vi "Login_Main P3.vi"() -> (3 "Login pass":bool)   [LabVIEW 2022 SP3]
uses:
  <vilib>/Utility/error.llb/Trim Whitespace One-Sided.vi
  Globals/Phase III Globals.vi
  <vilib>/Utility/file.llb/Read Delimited Spreadsheet (string).vi
  <vilib>/Utility/file.llb/Write Delimited Spreadsheet (string).vi
panel:
  in  "Enter":bool
  in  "Stop Button":bool
  out "Pass = True":bool
  in  "Change Password":bool
  in  "Show Password":bool
  in  "Password":string
  in  "Select User":u16(ring) items=["Vigneshwaran", "Kannan"]
  # "Agnikul Cosmos"
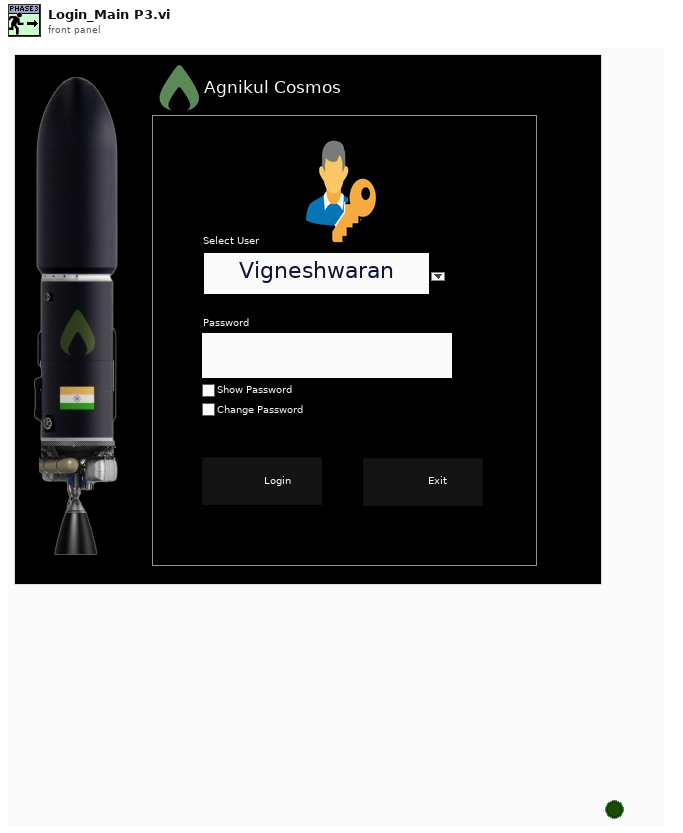
[diagram p1: front panel]
types:
  T1 = typedef "file folder ctl.ctl" = cluster{"Datalog path":path, "Configuration path":path, "Signal list path":path, "Sub vi's":path, "Authentication":path}
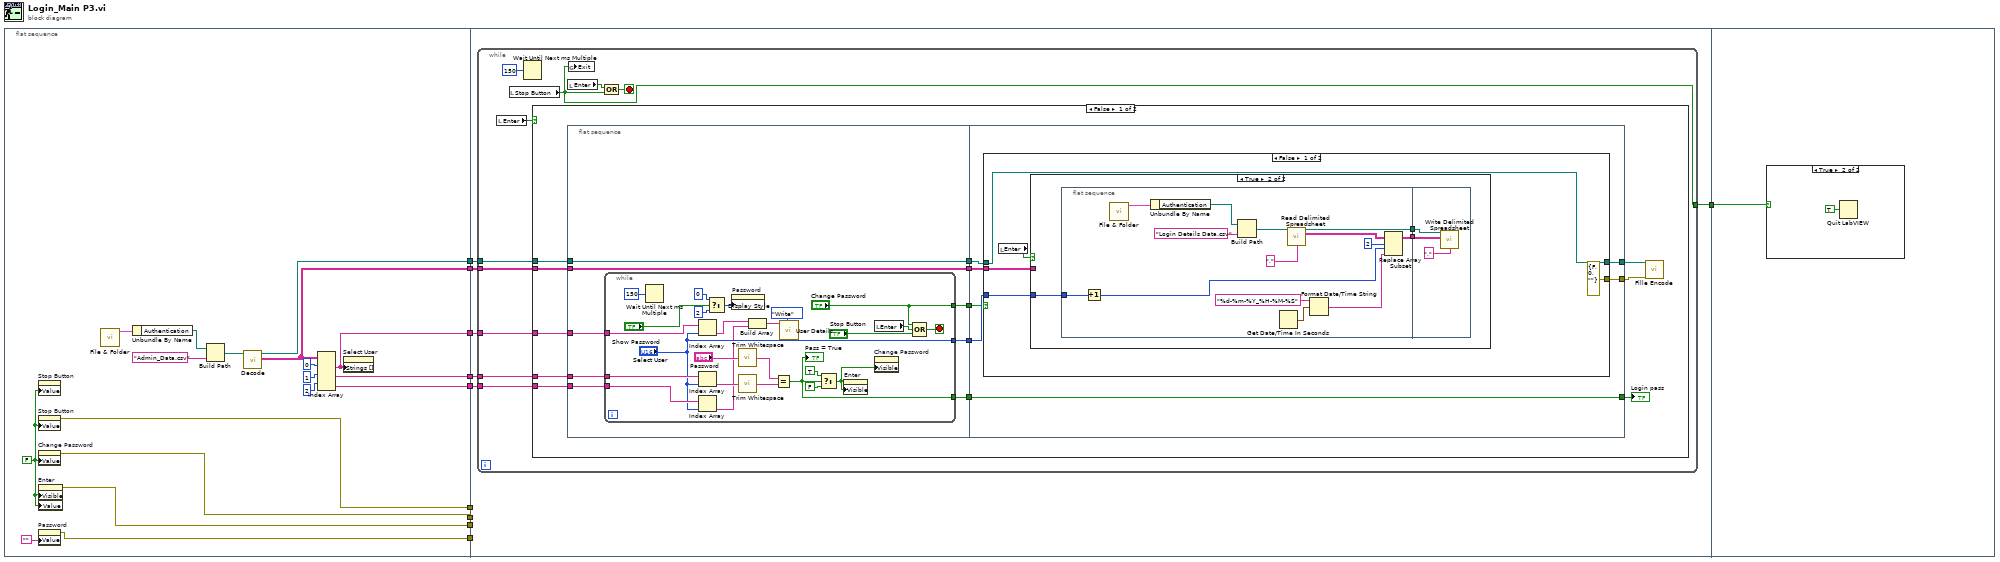
[diagram p0: block diagram]
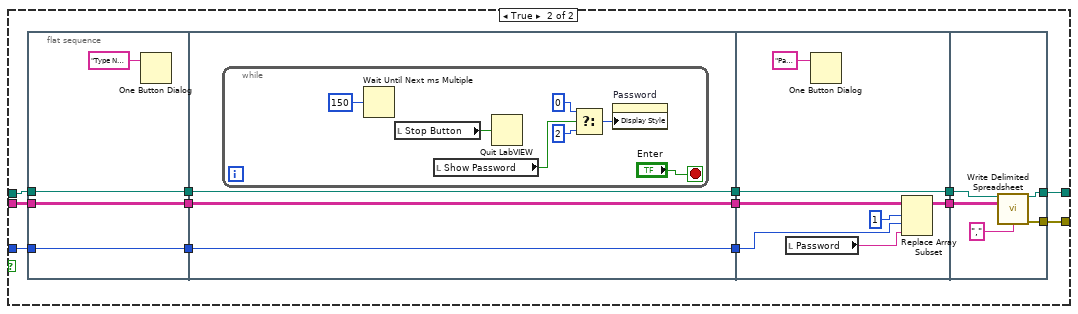
[diagram p3: hidden frame]
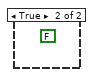
[diagram p4: hidden frame]
diagram:
  n1 = flat-sequence {
    tunnel: [w26] -> w10
    tunnel: [w11] -> w9
    tunnel: [w20] -> w8
    tunnel: [w25] -> w7
    tunnel: [w12] -> w6
    tunnel: [w22] -> w5
    tunnel: [w21] -> w4
    tunnel: [w19] -> w3
    tunnel: [w15] -> w2
    tunnel: w4 -> [_]
    tunnel: w5 -> [_]
    tunnel: w6 -> [w32]
    tunnel: w7 -> [_]
    tunnel: w8 -> [_]
    tunnel: w9 -> [w33]
    tunnel: w10 -> [w34]
    tunnel: w3 -> [w31]
    tunnel: w2 -> [w30]
    tunnel: [w29] -> w1
    tunnel: w1 -> [w162]
    frame #0 {
      w14 = FALSE ("Change Password")
      n2 = property on="Stop Button" class="Bool (strict)"("Value"=w14) -> ()  [unwired: 2 in, 2 out]
      n3 = property on="Stop Button" class="Bool (strict)"("Value"=w14) -> (error out=w21:errorcluster)  [unwired: 2 in, 1 out]
      n4 = property on="Change Password" class="Bool (strict)"("Value"=w14) -> (error out=w25:errorcluster)  [unwired: 2 in, 1 out]
      n5 = property on="Enter" class="Bool (strict)"("Visible"=w14, "Value"=w14) -> (error out=w20:errorcluster)  [unwired: 2 in, 1 out]
      n6 = property on="Password" class="Str"("Value"="") -> (error out=w22:errorcluster)  [unwired: 2 in, 1 out]
      n7 = call "File & Folder.vi"() -> ("File Output"=w18:T1)  [unwired: 10 in, 1 out]
      n8 = Unbundle By Name(w18) -> ("Authentication"=w17:path)
      n9 = Build Path(base path=w17, name or relative path="Admin_Data.csv" ("name")) -> (appended path=w13:path)
      n10 = call "Decode.vi"("Encoded  File"=w13) -> ("array"=w11:string[][], "Decoded File"=w12:path)  [unwired: 9 in]
      n11 = Index Array(array=w11, index (row) #1=0 ("index (row)"), index (row) #2=1 ("index (row)"), index (row) #3=2 ("disabled index (col)")) -> (element #1=w19:string[], element #2=w26:string[], element #3=w15:string[])  [unwired: 3 in]
      n12 = property on="Select User" class="Ring (strict)"("Strings []"=w19) -> ()  [unwired: 2 in, 2 out]
    }
    frame #1 {
      n13 = while {
        tunnel: w34 -> [w43]
        tunnel: w33 -> [w42]
        tunnel: w32 -> [w41]
        tunnel: w31 -> [w39]
        tunnel: w30 -> [w38]
        tunnel: [w35] -> w29
        stop <- w37 stop-if-true
        n14 = local read "Enter"() -> (w40:bool)
        n15 = local read "Stop Button"() -> (w35:bool)
        n16 = Wait Until Next ms Multiple(millisecond multiple=u32 150) -> ()  [unwired: 1 out]
        n17 = case shown="False" w40 {
          tunnel: w43 -> [w55 _]
          tunnel: w42 -> [w54 _]
          tunnel: w41 -> [w51 _]
          tunnel: w39 -> [w50 _]
          tunnel: w38 -> [w49 _]
          frame False {
            n18 = flat-sequence {
              tunnel: [w65] -> w57
              tunnel: [w64] -> w56
              tunnel: w54 -> [w65]
              tunnel: w55 -> [w63]
              tunnel: [w62] -> w53
              tunnel: [w61] -> w52
              tunnel: w51 -> [w61]
              tunnel: w50 -> [w60]
              tunnel: w49 -> [w59]
              tunnel: [w58] -> w48
              tunnel: w57 -> [w97]
              tunnel: w56 -> [w96]
              tunnel: w53 -> [w95]
              tunnel: w52 -> [w91]
              tunnel: w48 -> [w94]
              tunnel: [w94] -> w47
              tunnel: [w93] -> w46
              tunnel: [w92] -> w45
              frame #0 {
                n19 = while {
                  tunnel: ["Select User"] -> w64
                  tunnel: w63 -> [w90]
                  tunnel: ["Change Password"] -> w62
                  tunnel: w60 -> [w74]
                  tunnel: w59 -> [w73]
                  tunnel: [w70] -> w58
                  stop <- w79 stop-if-true
                  n20 = Wait Until Next ms Multiple(millisecond multiple=u32 150) -> ()  [unwired: 1 out]
                  n21 = Index Array(array=w74, index="Select User") -> (element=w68:string)
                  n22 = Index Array(array=w90, index="Select User") -> (element=w89:string)
                  n23 = Index Array(array=w73, index="Select User") -> (element=w67:string)
                  n24 = Select(t=u32 0 ("Display Style"), s="Show Password", f=u32 2 ("Display Style")) -> (s? t:f=w83:u32)
                  n25 = property on="Password" class="Str"("Display Style"=w83) -> ()  [unwired: 2 in, 2 out]
                  n26 = call <vilib>:"Trim Whitespace.vi"("string"="Password") -> ("trimmed string"=w85:string)  [unwired: 1 in]
                  n27 = call <vilib>:"Trim Whitespace.vi"("string"=w89) -> ("trimmed string"=w75:string)  [unwired: 1 in]
                  n28 = Build Array(w68, w67) -> (w66:string[])
                  n29 = Equal?(x=w85, y=w75) -> (x = y?=w70:bool)
                  "Pass = True" <- w70
                  n30 = call "User Details.vi"("Enum"=enum16{"Read", "Write"}."Write", "User details"=w66) -> ()  [unwired: 8 in, 2 out]
                  n31 = Select(t=TRUE, s=w70, f=FALSE ("Visible")) -> (s? t:f=w76:bool)
                  n32 = property on="Enter" class="Bool (strict)"("Visible"=w76) -> ()  [unwired: 2 in, 2 out]
                  n33 = local read "Enter"() -> (w77:bool)
                  n34 = property on="Change Password" class="Bool (strict)"("Visible"=w76) -> ()  [unwired: 2 in, 2 out]
                  n35 = Compound Arithmetic op=OR("Change Password", w77, "Stop Button") -> (w79:bool)
                }
              }
              frame #1 {
                n36 = case shown="False" w95 {
                  tunnel: w97 -> [w102 w133]
                  tunnel: w96 -> [w101 w130]
                  tunnel: w91 -> [w99 w125]
                  tunnel: [w99 w124] -> w93
                  tunnel: [errorcluster {"status"=FALSE, "code"=0, "source"=""} ("error out") w123] -> w92
                  frame False {
                    n37 = local read "Enter"() -> (w100:bool)
                    n38 = case shown="True" w100 {
                      tunnel: w102 -> [_ _]
                      tunnel: w101 -> [_ w105]
                      frame False {
                      }
                      frame True {
                        n39 = flat-sequence {
                          tunnel: w105 -> [w119]
                          tunnel: [w109] -> w104
                          tunnel: [w108] -> w103
                          tunnel: w104 -> [w121]
                          tunnel: w103 -> [w122]
                          frame #0 {
                            n40 = Increment(x=w119) -> (x+1=w112:u16)
                            n41 = call "File & Folder.vi"() -> ("File Output"=w115:T1)  [unwired: 10 in, 1 out]
                            n42 = Unbundle By Name(w115) -> ("Authentication"=w114:path)
                            n43 = Build Path(base path=w114, name or relative path="Login Details Data.csv" ("name")) -> (appended path=w111:path)
                            n44 = Get Date/Time In Seconds() -> (seconds since 1Jan1904=w106:timestamp)
                            n45 = call-poly <vilib>:"Read Delimited Spreadsheet.vi"("file path (dialog if empty)"=w111, "delimiter (\\t)"="," ("delimiter (\\t)")) -> ("new file path (Not A Path if cancelled)"=w108:path, "all rows"=w110:string[][])  [unwired: 8 in, 4 out]
                            n46 = Format Date/Time String(time format string (%c)="%d-%m-%Y_%H-%M-%S", seconds (now)=w106) -> (date/time string=w117:string)  [unwired: 1 in]
                            n47 = Replace Array Subset(array=w110, new element=w117, index (row)=2, index (col)=w112) -> (w109:string[][])
                          }
                          frame #1 {
                            n48 = call-poly <vilib>:"Write Delimited Spreadsheet.vi"("file path (dialog if empty)"=w122, "2D data"=w121, "delimiter (\\t)"="," ("delimiter (\\t)")) -> ()  [unwired: 11 in, 2 out]
                          }
                        }
                      }
                    }
                  }
                  frame True {
                    n49 = flat-sequence {
                      tunnel: [w139] -> w134
                      tunnel: w133 -> [w139]
                      tunnel: [w138] -> w131
                      tunnel: w130 -> [w138]
                      tunnel: [w137] -> w126
                      tunnel: w125 -> [w137]
                      tunnel: [w142] -> w135
                      tunnel: w134 -> [w142]
                      tunnel: [w141] -> w132
                      tunnel: w131 -> [w141]
                      tunnel: [w140] -> w127
                      tunnel: w126 -> [w140]
                      tunnel: w135 -> [w155]
                      tunnel: w132 -> [w153]
                      tunnel: [w151] -> w129
                      tunnel: [w150] -> w128
                      tunnel: w127 -> [w150]
                      tunnel: w129 -> [w161]
                      tunnel: w128 -> [w160]
                      tunnel: [w158] -> w124
                      tunnel: [w157] -> w123
                      frame #0 {
                        n50 = One Button Dialog(message="Type New Password and Press Enter button") -> ()  [unwired: 1 in, 1 out]
                      }
                      frame #1 {
                        n51 = while {
                          stop <- "Enter" stop-if-true
                          n52 = Wait Until Next ms Multiple(millisecond multiple=u32 150) -> ()  [unwired: 1 out]
                          n53 = local read "Stop Button"() -> (w148:bool)
                          n54 = local read "Show Password"() -> (w143:bool)
                          n55 = Quit LabVIEW(quit? (T)=w148) -> ()
                          n56 = Select(t=u32 0 ("Display Style"), s=w143, f=u32 2 ("Display Style")) -> (s? t:f=w144:u32)
                          n57 = property on="Password" class="Str"("Display Style"=w144) -> ()  [unwired: 2 in, 2 out]
                        }
                      }
                      frame #2 {
                        n58 = local read "Password"() -> (w152:string)
                        n59 = One Button Dialog(message="Password changed successfully, Please Login with new Password") -> ()  [unwired: 1 in, 1 out]
                        n60 = Replace Array Subset(array=w155, new element=w152, index (row)=1, index (col)=w153) -> (w151:string[][])
                      }
                      frame #3 {
                        n61 = call-poly <vilib>:"Write Delimited Spreadsheet.vi"("file path (dialog if empty)"=w160, "2D data"=w161, "delimiter (\\t)"="," ("delimiter (\\t)")) -> ("new file path (Not A Path if cancelled)"=w158:path, "error out"=w157:errorcluster)  [unwired: 11 in]
                      }
                    }
                  }
                }
              }
            }
            n62 = call "Fille Encode.vi"("error in"=w45, "Original File"=w46) -> ()  [unwired: 8 in, 2 out]
            "Login pass" <- w47
          }
          frame True {
            (unwired) FALSE
          }
        }
        n63 = local read "Enter"() -> (w36:bool)
        n64 = global write "Phase III Globals.vi" "Exit"(w35) -> ()
        n65 = Compound Arithmetic op=OR(w36, w35) -> (w37:bool)
      }
    }
    frame #2 {
      n66 = case shown="True" w162 {
        frame False {
        }
        frame True {
          n67 = Quit LabVIEW(quit? (T)=TRUE) -> ()
        }
      }
    }
  }
